vi "Initialize Actor.vi"(7 "Host Name":string, 8 "error in (no error)":errorcluster, 9 "Actor Name":string, 10 "Message Broker Interface":refnum<class "Message Broker Interface.lvclass">, 11 "Bank Account in":refnum<class "Bank Account.lvclass">) -> (0 "error out":errorcluster, 3 "Bank Account out":refnum<class "Bank Account.lvclass">)   [LabVIEW 2016, in "CLD Exam - ATM.lvlib" / "Bank Account.lvclass"]
uses:
  Bank Account.lvclass
  Mediator/Classes/Message Broker Interface/Message Broker Interface.lvclass
  Bank Account.lvclass/Bank Account.ctl
  Mediator/Classes/Message Transport Event/Message Transport Event.lvclass
  D:/Repos/Stream/software/Mediator/Classes/Message Transport Interface/Message Transport Interface.lvclass
  Mediator/Classes/Mediated Synchronous Actor/Mediated Synchronous Actor.lvclass
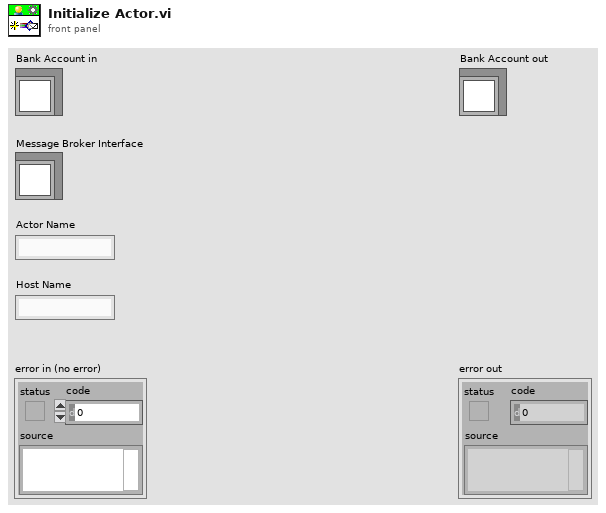
[diagram p1: front panel]
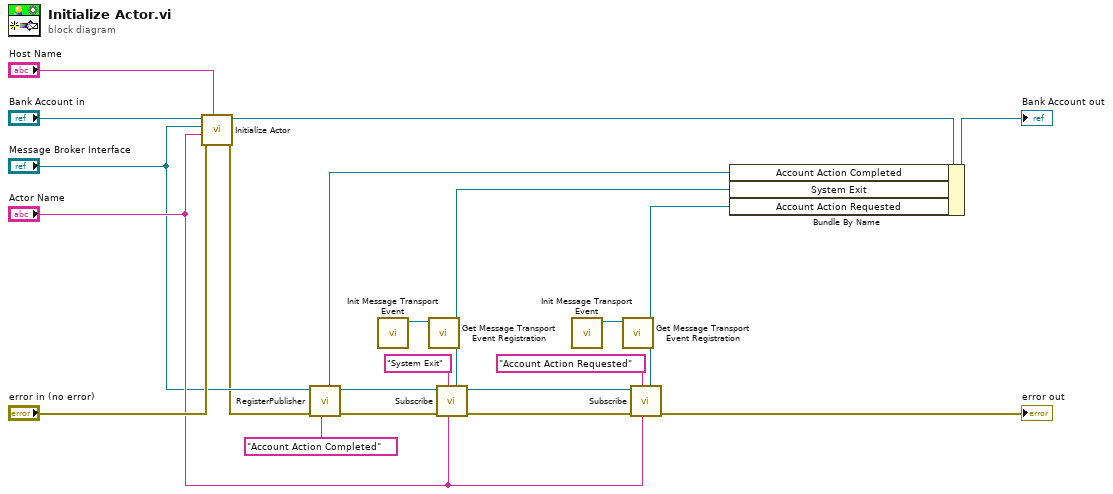
[diagram p0: block diagram]
diagram:
  n1 = call-parent "Initialize Actor.vi"("Host Name"="Host Name", "error in (no error)"="error in (no error)", "Actor Name"="Actor Name", "Message Broker Interface"="Message Broker Interface", "Mediated Synchronous Actor in"="Bank Account in") -> ("error out"=w5:errorcluster, "Mediated Synchronous Actor out"=w20:refnum<class "Bank Account.lvclass">)  [unwired: 5 in]
  n2 = call-dynamic "RegisterPublisher.vi"("Topic Name"="Account Action Completed", "error in (no error)"=w5, "Message Broker Interface in"="Message Broker Interface") -> ("error out"=w3:errorcluster, "Message Broker Interface out"=w4:refnum<class "Message Broker Interface.lvclass">, "Transport"=w9:refnum<class "Message Transport Queue.lvclass">)  [unwired: 4 in, 2 out]
  n3 = call "Init Message Transport Event.vi"() -> ("Message Transport Event out"=w12:refnum<class "Message Transport Event.lvclass">)  [unwired: 10 in, 1 out]
  n4 = call "Get Message Transport Event Registration.vi"("Message Transport Event in"=w12) -> ("Event Registration Refnum"=w8:refnum<event-registration>, "Message Transport Event out"=w13:refnum<class "Message Transport Event.lvclass">)  [unwired: 7 in, 2 out]
  n5 = call-dynamic "Subscribe.vi"("Message Transport Interface"=w13, "Subscriber Name"="Actor Name", "Topic Name"="System Exit", "error in (no error)"=w3, "Message Broker Interface in"=w4) -> ("error out"=w1:errorcluster, "Message Broker Interface out"=w2:refnum<class "Message Broker Interface.lvclass">)  [unwired: 4 in, 1 out]
  n6 = call "Init Message Transport Event.vi"() -> ("Message Transport Event out"=w15:refnum<class "Message Transport Event.lvclass">)  [unwired: 10 in, 1 out]
  n7 = call "Get Message Transport Event Registration.vi"("Message Transport Event in"=w15) -> ("Event Registration Refnum"=w7:refnum<event-registration>, "Message Transport Event out"=w16:refnum<class "Message Transport Event.lvclass">)  [unwired: 7 in, 2 out]
  n8 = call-dynamic "Subscribe.vi"("Message Transport Interface"=w16, "Subscriber Name"="Actor Name", "Topic Name"="Account Action Requested", "error in (no error)"=w1, "Message Broker Interface in"=w2) -> ("error out"=→"error out":errorcluster)  [unwired: 4 in, 2 out]
  n9 = Bundle By Name(cluster=w20, "Account Action Completed"=w9, "System Exit"=w8, "Account Action Requested"=w7) -> (→"Bank Account out":refnum<class "Bank Account.lvclass">)
